vi "General VISA transaction.vi"(6 "Wait For SRQ":bool, 7 "Wait (mS)":dbl, 8 "error in (no error)":errorcluster, 9 "Command String":string, 10 "Eng Units?":bool, 11 "VISA Session":refnum<visa-resource-name>) -> (0 "error out":errorcluster, 1 "String Resonse":string, 2 "Measurement":dbl[](array[numeric]), 3 "dup VISA Session":refnum<visa-resource-name>, 4 "Stop":bool, 5 "Read ∆ Time":dbl)   [LabVIEW 2020]
doc: "This VI sends a Command String and reads the response. All numbers are extracted from the response and returned in the data array.. If no reading is obtained a single zero is returned.\nScott Hannahs, <sth@magnet.fsu.edu> NHMFL-FSU, May 2003"
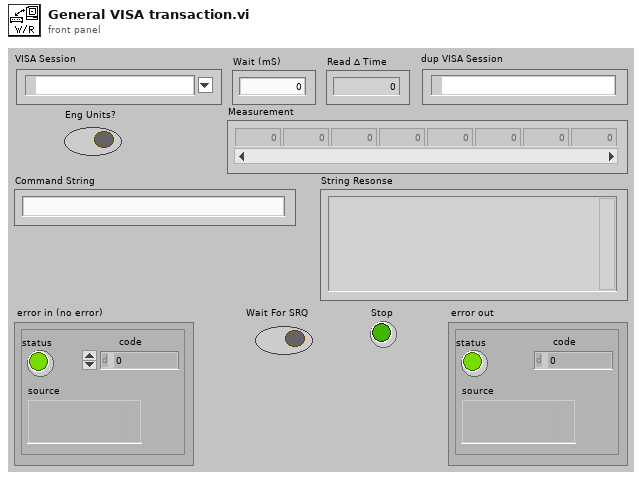
[diagram p1: front panel]
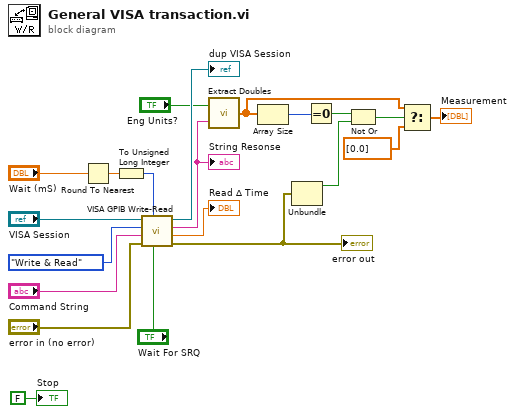
[diagram p0: block diagram]
diagram:
  n1 = Round To Nearest(number="Wait (mS)") -> (nearest integer value=w2:dbl)
  n2 = To Unsigned Long Integer(number=w2) -> (unsigned 32bit integer=w1:u32)
  n3 = call "VISA GPIB Write-Read.vi"("Wait For SRQ"="Wait For SRQ", "Wait (ms)"=w1, "error in (no error)"="error in (no error)", "Command"="Command String", "Action"=enum16{"Write", "Read", "Write & Read"}."Write & Read", "VISA resource name"="VISA Session") -> ("error out"=w12:errorcluster, "Read ∆ Time"=→"Read ∆ Time":dbl, "String Returned"=w13:string, "dup VISA Session"=→"dup VISA Session":refnum<visa-resource-name>)  [unwired: 2 in]
  "String Resonse" <- w13
  "error out" <- w12
  n4 = call "Extract Doubles.vi"("String"=w13, "Eng Units?"="Eng Units?") -> ("Data"=w16:dbl[])
  n5 = Array Size(array=w16) -> (size(s)=w20:i32)
  n6 = Unbundle(w12) -> ("status"=w18:bool)  [unwired: 2 out]
  n7 = Equal To 0?(x=w20) -> (x = 0?=w19:bool)
  n8 = Not Or(1:w18, 2:w19) -> (0:w17:bool)
  n9 = Select(t=w16, s=w17, f=dbl[] [0.0]) -> (s? t:f=→"Measurement":dbl[])
  "Stop" <- FALSE
